vi "create transfer specification.vi"(8 "error in":errorcluster, 9 "mapping specification":T3[](array[typedef]), 10 "data dictionary source in":refnum<class "data dictionary.lvclass">, 11 "data dictionary sink in":refnum<class "data dictionary.lvclass">) -> (0 "error out":errorcluster, 1 "transfer specification":T1[](array[typedef]), 2 "data dictionary source out":refnum<class "data dictionary.lvclass">, 3 "data dictionary sink out":refnum<class "data dictionary.lvclass">)   [LabVIEW 2013, in "tag bus.lvlib" / "data dictionary.lvclass"]
doc: "Uses two data dictionaries and a set of tag names and types to create a transfer specification. This transfer specification can be used to move data from one table to another table. These tables do not need to share the same tags."
uses:
  data dictionary.lvclass
  table/mapping specification.ctl
  tag/Data Type.ctl
  table/mapping.ctl
  table/transfer specification.ctl
  tag/tag descriptor.lvclass
  table/data table.lvlib
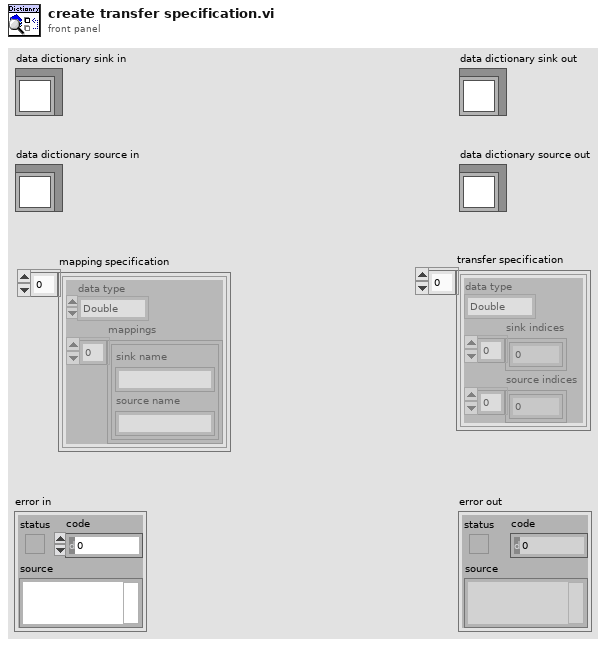
[diagram p1: front panel]
types:
  T1 = typedef "tag bus.lvlib/data table.lvlib/transfer specification.ctl" = cluster{"data type":T2, "sink indices":i32[], "source indices":i32[]}
  T2 = typedef "tag bus.lvlib/tag descriptor.lvclass/Data Type.ctl" = enum16{"Double", "Single", "I64", "I32", "I16", "I8", "U64", "U32", "U16", "U8", "Boolean", "String", "Array of Double", "Array of Single", "Array of I64", "Array of I32", "Array of I16", "Array of I8", "Array of U64", "Array of U32", "Array of U16", "Array of U8", "Array of Boolean", "Array of String"}
  T3 = typedef "tag bus.lvlib/data table.lvlib/mapping specification.ctl" = cluster{"data type":T2, "mappings":T4[]}
  T4 = typedef "tag bus.lvlib/data table.lvlib/mapping.ctl" = cluster{"sink name":string, "source name":string}
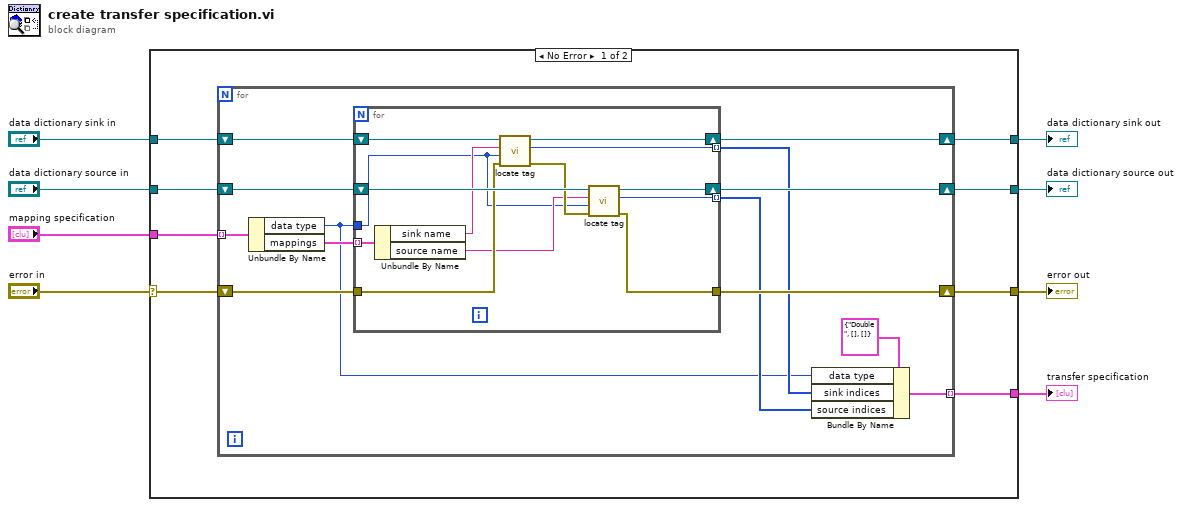
[diagram p0: block diagram]
diagram:
  n1 = case shown="No Error" "error in" {
    selector: "error in" -> [w11 w45]
    tunnel: [w10 w45] -> w7
    tunnel: [w15 w44] -> w5
    tunnel: "data dictionary sink in" -> [w16 w44]
    tunnel: "data dictionary source in" -> [w14 w43]
    tunnel: "mapping specification" -> [w12 _]
    tunnel: [w13 w43] -> w2
    tunnel: [w9 _] -> w1
    frame No Error {
      n2 = for {
        tunnel: w12 -> [w29] mode=indexing
        shift-right: [w23] -> w10
        shift-left: w11 -> [w24]
        tunnel: [w17] -> w9 mode=indexing
        shift-right: [w27] -> w15
        shift-left: w16 -> [w28]
        shift-right: [w25] -> w13
        shift-left: w14 -> [w26]
        n3 = Unbundle By Name(w29) -> ("data type"=w18:T2, "mappings"=w22:T4[])
        n4 = for {
          tunnel: w24 -> [w38]
          tunnel: [w36] -> w23
          tunnel: w22 -> [w35] mode=indexing
          tunnel: w18 -> [w30]
          tunnel: [w32] -> w20 mode=indexing
          tunnel: [w31] -> w19 mode=indexing
          shift-right: [w41] -> w27
          shift-left: w28 -> [w42]
          shift-right: [w39] -> w25
          shift-left: w26 -> [w40]
          n5 = Unbundle By Name(w35) -> ("sink name"=w34:string, "source name"=w33:string)
          n6 = call "locate tag.vi"("error in"=w38, "data type"=w30, "name"=w34, "data dictionary in"=w42) -> ("error out"=w37:errorcluster, "index"=w32:i32, "data dictionary out"=w41:refnum<class "data dictionary.lvclass">)  [unwired: 5 in]
          n7 = call "locate tag.vi"("error in"=w37, "data type"=w30, "name"=w33, "data dictionary in"=w40) -> ("error out"=w36:errorcluster, "index"=w31:i32, "data dictionary out"=w39:refnum<class "data dictionary.lvclass">)  [unwired: 5 in]
        }
        n8 = Bundle By Name(cluster=T1 {"data type"=enum."Double", "sink indices"=[], "source indices"=[]} ("merge specification"), "data type"=w18, "sink indices"=w20, "source indices"=w19) -> (w17:T1)
      }
    }
    frame Error {
    }
  }
  "error out" <- w7
  "data dictionary sink out" <- w5
  "data dictionary source out" <- w2
  "transfer specification" <- w1
